vi "Configure Voltage Source.vi"(0 "VISA resource name":refnum<visa-resource-name>, 1 "Enable Voltage Source (F: Disable)":bool, 2 "Enable Interlock (F: Disable)":bool, 5 "Voltage Source Range (10 V)":u16(ring)=10 items=["10 V"=10, "50 V"=50, "500 V"=500], 7 "Voltage Level (0 V)":dbl, 9 "Current Limit (25 mA)":u16(ring) items=["25 mA", "2.5 mA", "250 uA", "25 uA"], 11 "error in (no error)":errorcluster) -> (4 "VISA resource name out":refnum<visa-resource-name>, 15 "error out":errorcluster)   [LabVIEW 2020, in "Keithley 648X Series.lvlib"]
doc: "Configures the voltage source. The voltage source is used by the instrument in making resistance calculations.\n\n<b>Note:</b>\nThis supports Model 6487 only"
uses:
  <instrlib>/Keithley 648X Series/Keithley 648X Series.lvlib
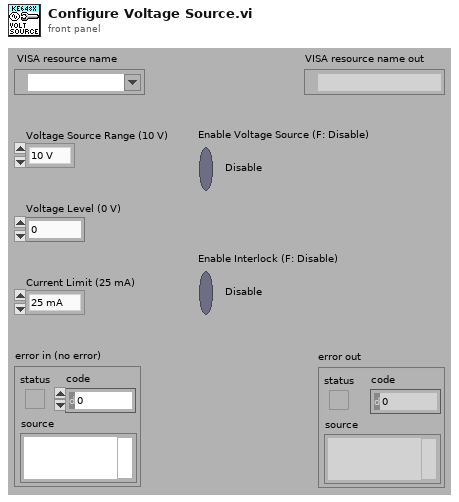
[diagram p1: front panel]
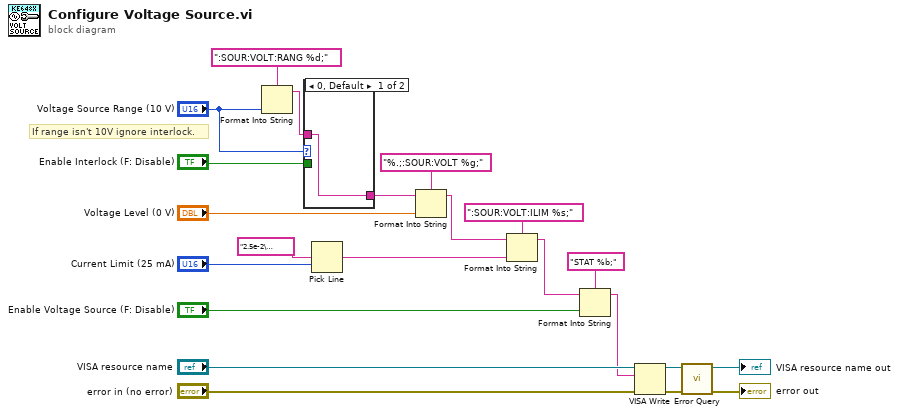
[diagram p0: block diagram]
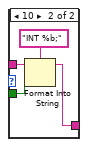
[diagram p2: hidden frame]
diagram:
  # "If range isn't 10V ignore interlock."
  n1 = Format Into String(format string=":SOUR:VOLT:RANG %d;", "Voltage Source Range (10 V)") -> (resulting string=w15:string)  [unwired: 2 in, 1 out]
  n2 = case shown="0, Default" "Voltage Source Range (10 V)" {
    tunnel: w15 -> [w23 w26]
    tunnel: [w23 w25] -> w12
    tunnel: "Enable Interlock (F: Disable)" -> [_ w24]
    frame 0, Default {
    }
    frame 10 {
      n3 = Format Into String(format string="INT %b;", initial string=w26, w24) -> (resulting string=w25:string)  [unwired: 1 in, 1 out]
    }
  }
  n4 = Pick Line(multi-line string="2.5e-2\n2.5e-3\n2.5e-4\n2.5e-5", line index="Current Limit (25 mA)") -> (output string=w9:string)  [unwired: 1 in]
  n5 = Format Into String(format string="%.;:SOUR:VOLT %g;", initial string=w12, "Voltage Level (0 V)") -> (resulting string=w7:string)  [unwired: 1 in, 1 out]
  n6 = Format Into String(format string=":SOUR:VOLT:ILIM %s;", initial string=w7, w9) -> (resulting string=w4:string)  [unwired: 1 in, 1 out]
  n7 = Format Into String(format string="STAT %b;", initial string=w4, "Enable Voltage Source (F: Disable)") -> (resulting string=w3:string)  [unwired: 1 in, 1 out]
  n8 = VISA Write(VISA resource name="VISA resource name", write buffer=w3, error in (no error)="error in (no error)") -> (VISA resource name out=w18:refnum<visa-resource-name>, error out=w17:errorcluster)  [unwired: 1 out]
  n9 = call <instrlib>:"Error Query.vi"("error in (no error)"=w17, "VISA resource name"=w18) -> ("error out"=→"error out":errorcluster, "VISA resource name out"=→"VISA resource name out":refnum<visa-resource-name>)  [unwired: 6 in, 2 out]
